vi "Insert JSON Element.vi"(8 "error in (no error)":errorcluster, 9 "VElement":variant, 10 "VCluster parent":variant, 11 "Parent Cluster Name":string) -> (0 "error out":errorcluster, 3 "VCluster":variant)   [LabVIEW 2015]
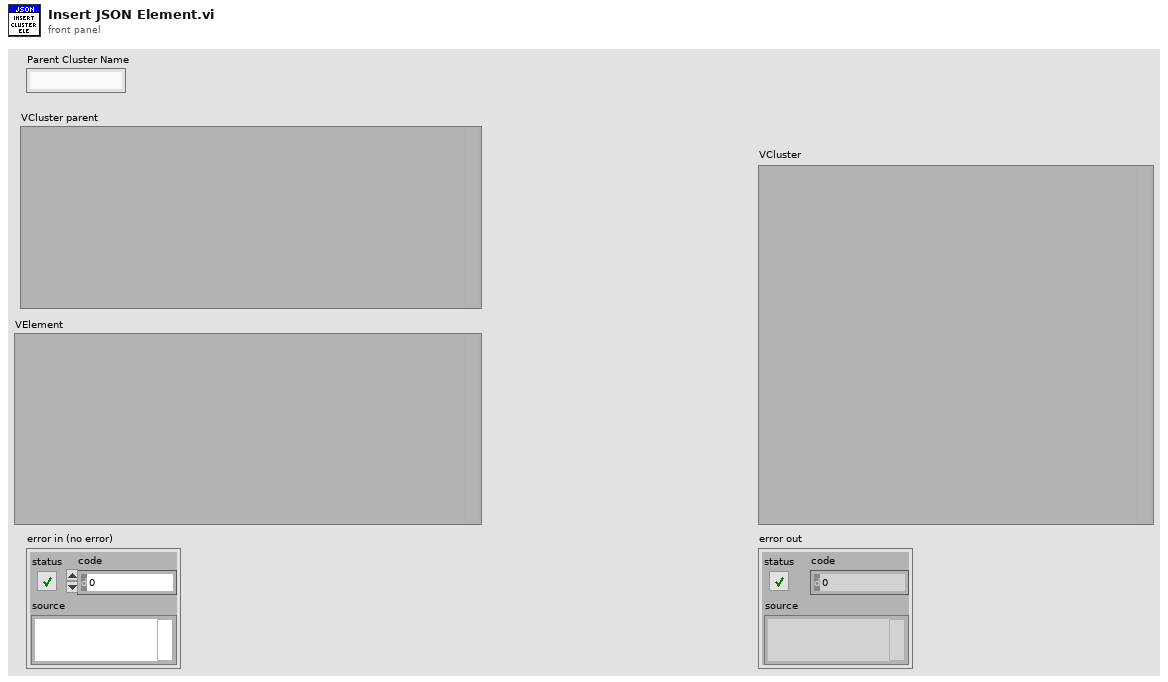
[diagram p1: front panel]
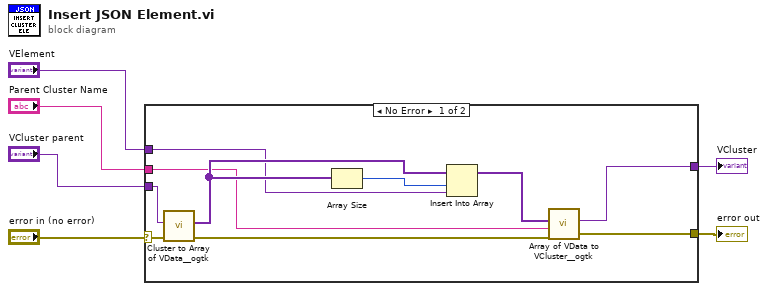
[diagram p0: block diagram]
diagram:
  n1 = case shown="No Error" "error in (no error)" {
    selector: "error in (no error)" -> [w12 w17]
    tunnel: "Parent Cluster Name" -> [w10 _]
    tunnel: "VElement" -> [w9 _]
    tunnel: "VCluster parent" -> [w11 w18]
    tunnel: [w7 w18] -> w3
    tunnel: [w8 w17] -> w2
    frame No Error {
      n2 = call <userlib>:"Cluster to Array of VData__ogtk.vi"("error in (no error)"=w12, "Cluster"=w11) -> ("error out"=w13:errorcluster, "Array of VData"=w14:variant[])  [unwired: 8 in]
      n3 = Array Size(array=w14) -> (size(s)=w15:i32)
      n4 = Insert Into Array(array=w14, index=w15, new element=w9) -> (w16:variant[])
      n5 = call <userlib>:"Array of VData to VCluster__ogtk.vi"("error in (no error)"=w13, "Cluster Name"=w10, "Array"=w16) -> ("error out"=w8:errorcluster, "VCluster"=w7:variant)  [unwired: 7 in]
    }
    frame Error {
    }
  }
  "VCluster" <- w3
  "error out" <- w2
